vi "lookup_table_and_invert.vi"() -> ()   [LabVIEW 2020]
doc: "VI che calcola l'istogramma dell'immagine"
uses:
  <vilib>/vision/NI_Vision_Development_Module.lvlib
panel:
  in  "Tab Control":enum32{"Immagini", "Istogrammi"}(tab)
  out "Gray level image":T1(plugin-control)
  out "Lookup":T1(plugin-control)
  in  "Operator":T2(ring)
  out "Invert":T1(plugin-control)
  in  "stop":bool
  in  "X Value":sgl format="%.2f"
  in  "Path Image Load":path
  in  "OK Button":bool
  in  "Path Save Image Invert":path
  in  "error in (no error)":errorcluster
  out "error out":errorcluster
  in  "Path Save Image LUT":path
  in  "OK Button 2":bool
  out "Istogramma":T3(graph)
  out "Istogramma Lookup":T3(graph)
  out "Istogramma Invert":T3(graph)
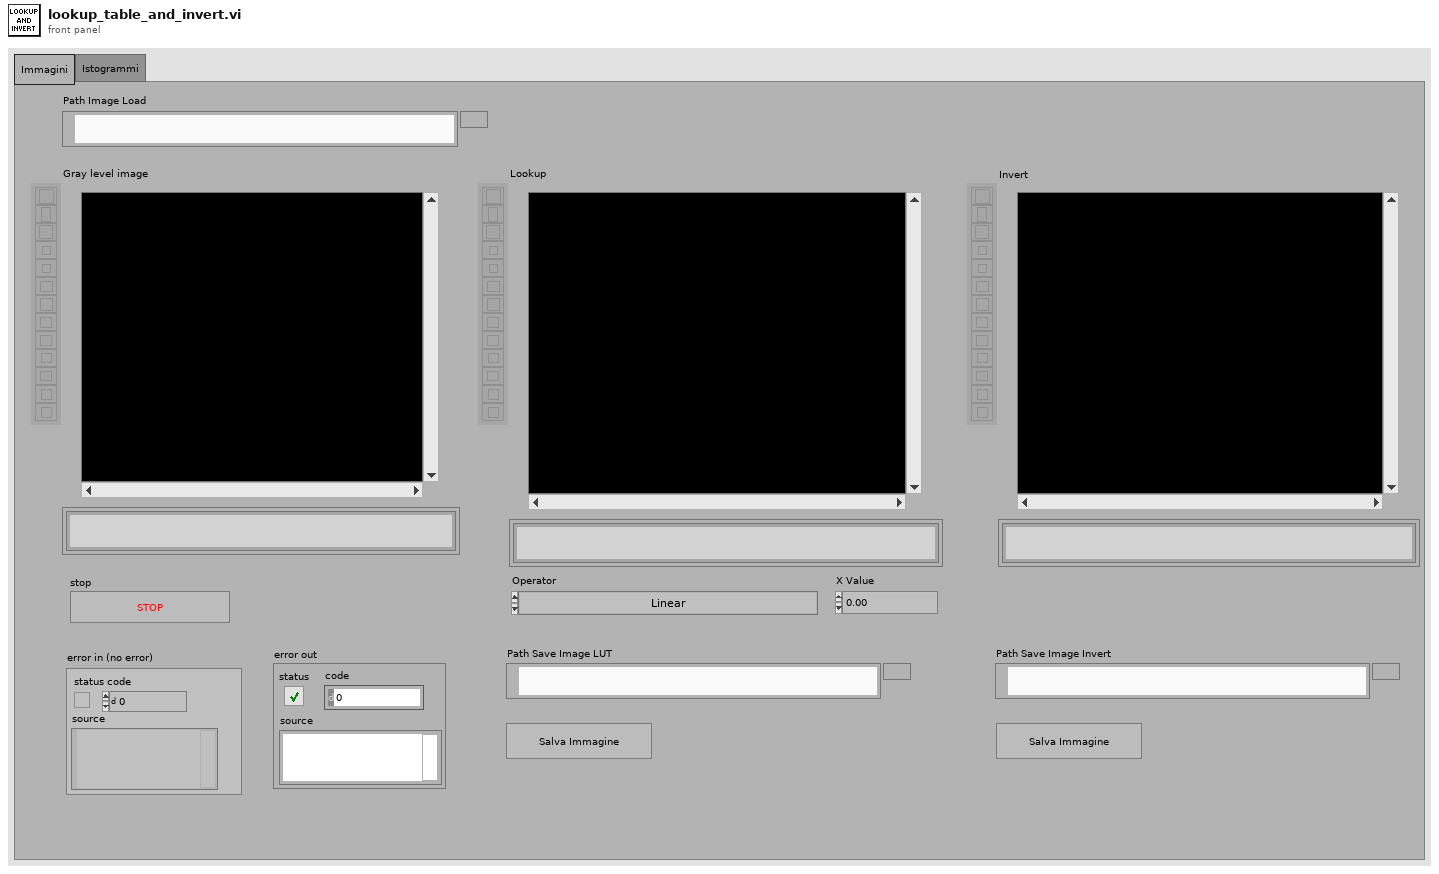
[diagram p1: front panel]
types:
  T1 = typedef "IMAQ Image.ctl" = refnum<image>
  T2 = enum32{"Linear", "Log", "Exp", "Square", "Square root", "Power X", "Power 1/X"}
  T3 = cluster{"Starting Value":sgl, "Incremental Value":sgl, "Histogram":u32[]}
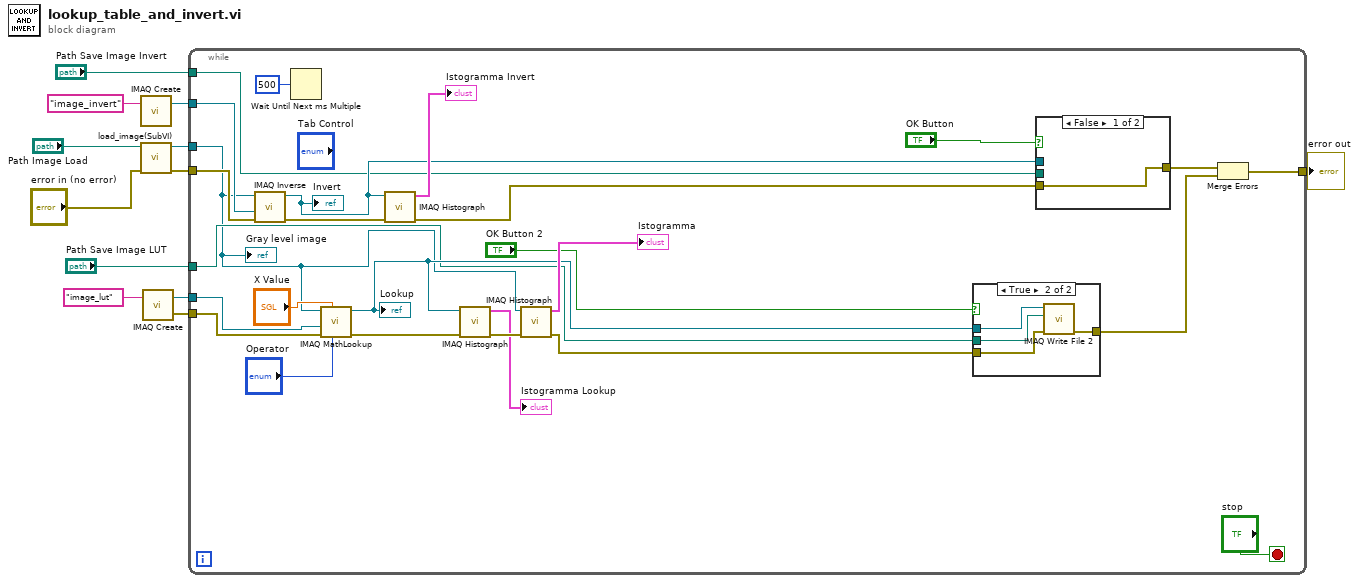
[diagram p0: block diagram]
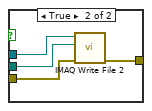
[diagram p3: hidden frame]
diagram:
  n1 = call "IMAQ Create"("Image Name"="image_invert") -> ("New Image"=w11:T1)  [unwired: 4 in, 1 out]
  n2 = call "load_image(SubVI).vi"("error in (no error)"="error in (no error)", "Image Path"="Path Image Load") -> ("error out"=w1:errorcluster, "Image GRAY"=w2:T1)  [unwired: 8 in]
  n3 = call "IMAQ Create"("Image Name"="image_lut") -> ("New Image"=w9:T1, "error out"=w8:errorcluster)  [unwired: 4 in]
  n4 = while {
    tunnel: w11 -> [w31]
    tunnel: w2 -> [w13]
    tunnel: "Path Save Image Invert" -> [w27]
    tunnel: w1 -> [w24]
    tunnel: w9 -> [w22]
    tunnel: w8 -> [w21]
    tunnel: [w19] -> w7
    tunnel: "Path Save Image LUT" -> [w16]
    stop <- "stop" stop-if-true
    n5 = call "IMAQ Inverse"("error in (no error)"=w24, "Image Dst"=w31, "Image Src"=w13) -> ("error out"=w26:errorcluster, "Image Dst Out"=w28:T1)  [unwired: 7 in]
    "Invert" <- w28
    n6 = Wait Until Next ms Multiple(millisecond multiple=u32 500) -> ()  [unwired: 1 out]
    n7 = call "IMAQ MathLookup"("Operator"="Operator", "X Value"="X Value", "error in (no error)"=w21, "Image Dst"=w22, "Image Src"=w13) -> ("error out"=w35:errorcluster, "Image Dst Out"=w18:T1)  [unwired: 5 in]
    "Lookup" <- w18
    n8 = call "IMAQ Histograph"("error in (no error)"=w26, "Image"=w28) -> ("error out"=w25:errorcluster, "Histogram Graph"=→"Istogramma Invert":T3)  [unwired: 6 in, 2 out]
    n9 = call "IMAQ Histograph"("error in (no error)"=w35, "Image"=w18) -> ("error out"=w34:errorcluster, "Histogram Graph"=→"Istogramma Lookup":T3)  [unwired: 6 in, 2 out]
    n10 = call "IMAQ Histograph"("error in (no error)"=w34, "Image"=w13) -> ("error out"=w15:errorcluster, "Histogram Graph"=→"Istogramma":T3)  [unwired: 6 in, 2 out]
    n11 = case shown="True" "OK Button 2" {
      tunnel: [w39 w43] -> w14
      tunnel: w16 -> [_ w42]
      tunnel: w18 -> [_ w41]
      tunnel: w15 -> [w39 w40]
      frame False {
      }
      frame True {
        n12 = call-poly "IMAQ Write File 2"("error in (no error)"=w40, "File Path"=w42, "Image"=w41) -> ("error out"=w43:errorcluster)  [unwired: 7 in, 1 out]
      }
    }
    n13 = case shown="False" "OK Button" {
      tunnel: w25 -> [w44 w48]
      tunnel: [w44 w47] -> w20
      tunnel: w27 -> [_ w46]
      tunnel: w28 -> [_ w45]
      frame False {
      }
      frame True {
        n14 = call-poly "IMAQ Write File 2"("error in (no error)"=w48, "File Path"=w46, "Image"=w45) -> ("error out"=w47:errorcluster)  [unwired: 7 in, 1 out]
      }
    }
    n15 = Merge Errors(w20, w14) -> (w19:errorcluster)
    "Gray level image" <- w13
  }
  "error out" <- w7
